vi "R45_2-RT.vi"() -> ()   [LabVIEW 2016]
uses:
  control vi/controls/Faraday cup states.ctl
  control vi/controls/Aperture states.ctl
  control vi/controls/Glassman Control.ctl
  SCA/controls/GP307 cluster.ctl
  <vilib>/FPGAPlugInAG/cRIO-9074/niLvFpga_Open_cRIO-9074.vi
  <vilib>/Utility/error.llb/Error Cluster From Error Code.vi
  <vilib>/rvi/errors/niLvFpgaAdjustHostInterfaceError.vi
  <vilib>/functionblocks/Control/PID/PID.vi
  <vilib>/rvi/interface/nirviOpenFPGA/nirviOpenFPGA.xnode
  Builds/cRIOs/R45-2-cRIO/FPGA/Controlsoftware2_FPGATarget8_R45crio2fpga_v8BgrifJ-aU.lvbitx
  R45_2-FPGA.vi
  <vilib>/rvi/interface/nirviReadWriteControl/nirviReadWriteControl.xnode
  control vi/controls/Glassman Readback.ctl
  control vi/controls/Aperture Readback.ctl
  control vi/controls/Faraday Cup Readback.ctl
  <vilib>/functionblocks/FB Core/FB Core.xnode
  <vilib>/functionblocks/NI_FunctionBlock Libraries.lvlib
  NiFpgaLv.dll
  <vilib>/NI_Real-Time Target Support.lvlib
panel:
  in  "Tab Control":T1(tab)
  out "R45 ExB 1 voltage set":dbl
  out "ExB 1- I read":dbl
  out "ExB 1- V read":dbl
  out "ExB 2+ I read":dbl
  out "ExB 2+ V read":dbl
  out "ExB 2- I read":dbl
  out "ExB 2- V read":dbl
  out "R45 ExB 2 voltage set":dbl
  out "ExB 1+ I read":dbl
  out "ExB 1+ V read":dbl
  out "GFM magnet current set":dbl
  out "GFM read string":string
  in  "output high - GFM":dbl=205.0
  in  "output low - GFM":dbl
  out "GFM field read":u8[](array[numeric])
  out "GFM field":dbl format="%#_8f"
  out "GFM command":u8[](array[numeric])
  out "R45 ExB 2 command string":string
  out "R45 ExB 2 command array":u8[](array[numeric])
  out "ExB #2 magnet current set":dbl
  out "GFM command string":string
  out "GFM field set":dbl
  out "ExB #1 magnet current set":dbl
  out "R45 ExB 1 command string":string
  out "R45 ExB 1 command array":u8[](array[numeric])
  out "proportional gain (Kc) - GFM":dbl
  out "integral time (Ti, min) - GFM":dbl
  out "derivative time (Td, min) - GFM":dbl
  out "Ion Gauge 3-2":u8[](array[numeric])
  out "Convectron gauge 3-2":u8[](array[numeric])
  out "Ion gauge 2-2":u8[](array[numeric])
  out "Ion gauge 2-1":u8[](array[numeric])
  out "Convectron 3-1":u8[](array[numeric])
  out "Ion gauge 3-1":u8[](array[numeric])
  out "Convectron 2-2":u8[](array[numeric])
  out "Convectron 2-1":u8[](array[numeric])
  out "Ion Gauge 4-1":u8[](array[numeric])
  out "Convectron Gauge 4-1":u8[](array[numeric])
  out "Ion Gauge 4-2":u8[](array[numeric])
  out "Convectron Gauge 4-2":u8[](array[numeric])
  out "R45 Quad  vac gauge cluster":T2
  out "R45 Detector vac gauge cluster":T2
  out "R45 ExB Slot vac gauge cluster":T2
  out "Detector FC status":T3
  out "Detector Aperture status":T4
  out "Detector Aperture Position":cluster{"IN sensor":bool, "OUT sensor":bool}
  out "Detector FC Position":cluster{"IN sensor":bool, "OUT sensor":bool}
  out "R45 Detector FC insert":bool
  out "R45 Detector Aperture insert":bool
  out "HV control loop error":errorcluster
  out "HV readback loop error":errorcluster
  out "Error Reporter":errorcluster
  out "ExB 1 PS loop error":errorcluster
  out "ExB 2 PS loop error":errorcluster
  out "GFM loop error":errorcluster
  out "Vacuum readback error":errorcluster
  out "Actuator loop error":errorcluster
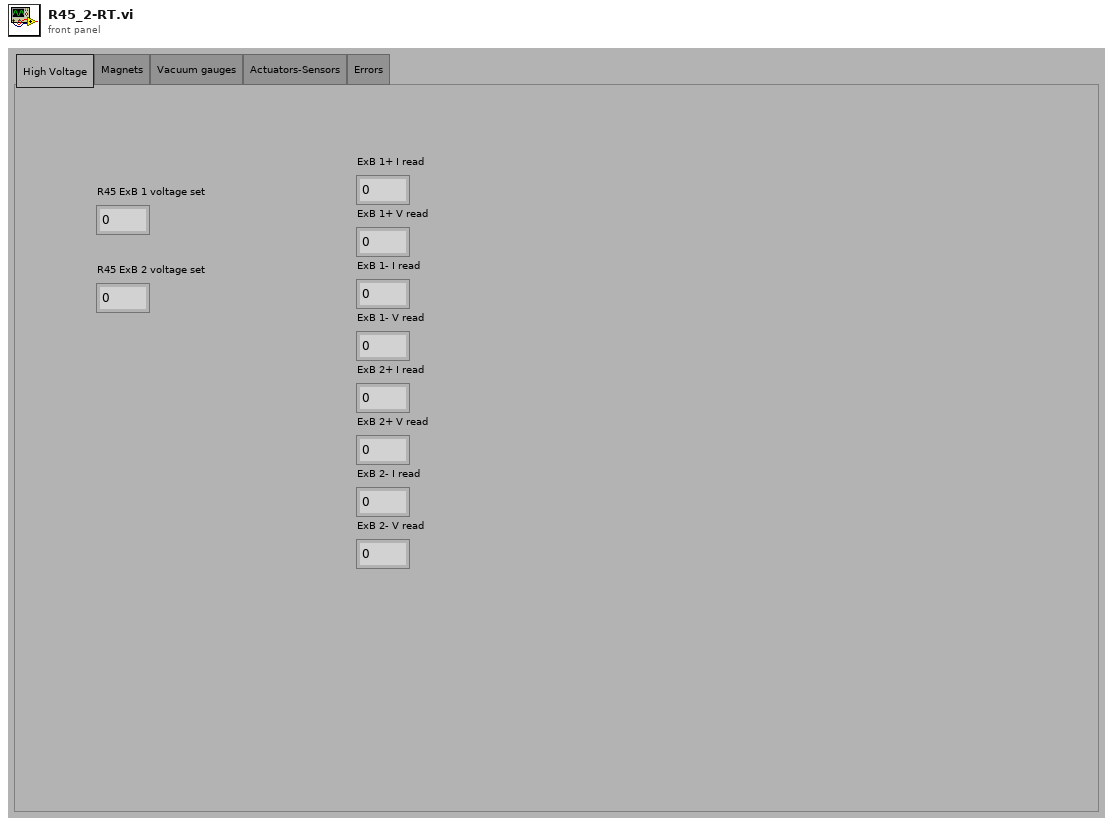
[diagram p1: front panel]
types:
  T1 = enum32{"High Voltage", "Magnets", "Vacuum gauges", "Actuators-Sensors", "Errors"}
  T2 = cluster{"Ion gauge 1":string, "Convectron  Gauge 1 ":string, "Ion Gauge 2":string, "Convectrom Gauge 2":string}
  T3 = typedef "Faraday cup states.ctl" = enum16{"FC status unclear", "FC in", "FC out"}
  T4 = typedef "Aperture states.ctl" = enum16{"Aperture status unclear", "Aperture in", "Aperture out"}
  T5 = typedef "Glassman Control.ctl" = cluster{"V-program":fxp<+/-,16,5>, "HV Enable":bool}
  T6 = typedef "Glassman Readback.ctl" = cluster{"I-monitor":fxp<+/-,16,5>, "V-monitor":fxp<+/-,16,5>}
  T7 = typedef "Aperture Readback.ctl" = cluster{"IN sensor":bool, "OUT sensor":bool}
  T8 = typedef "Faraday Cup Readback.ctl" = cluster{"IN sensor":bool, "OUT sensor":bool}
  T9 = typedef "GP307 cluster.ctl" = cluster{"Ion gauge 1":string, "Convectron  Gauge 1 ":string, "Ion Gauge 2":string, "Convectrom Gauge 2":string}
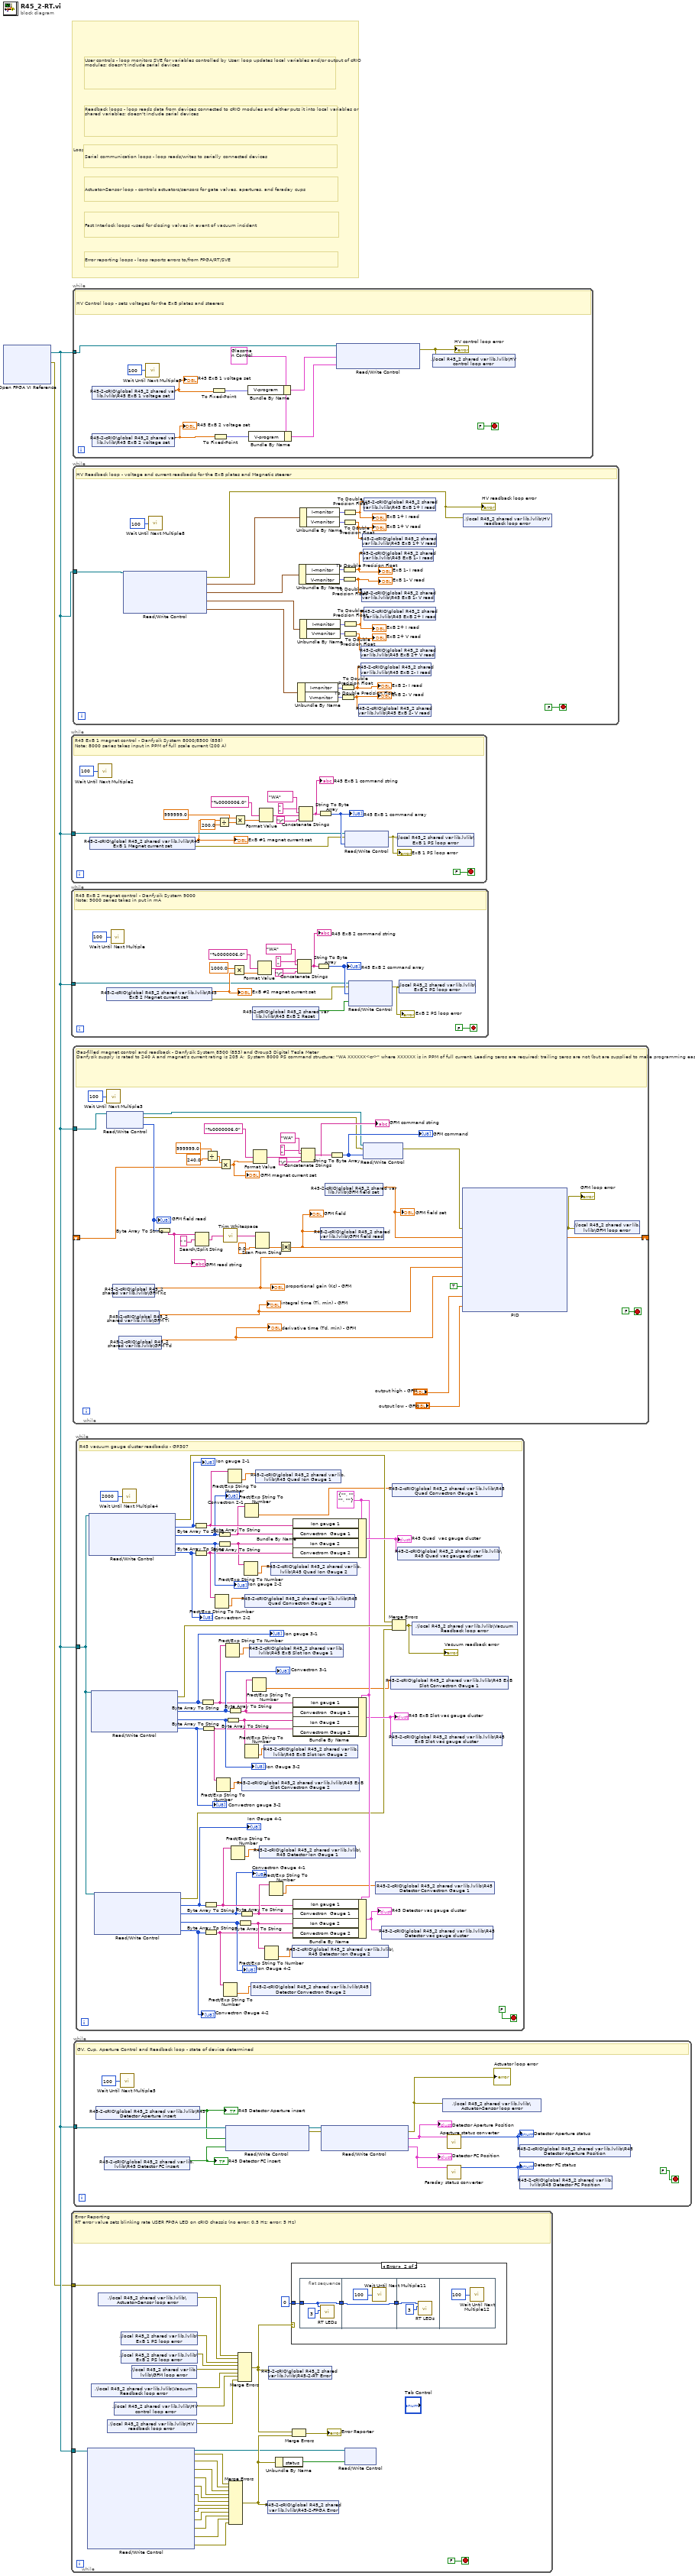
[diagram p0: block diagram]
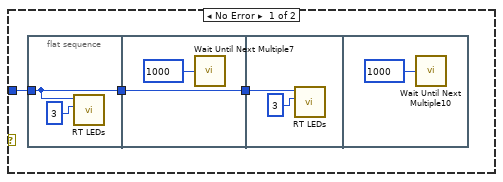
[diagram p2: hidden frame]
diagram:
  # "Serial communication loops - loop reads/writes to serially connected devices"
  # "Actuator-Sensor loop - controls actuators/sensors for gate valves, apertures, and faraday cups"
  # "Fast Interlock loops -used for closing valves in event of vacuum incident"
  # "Error reporting loops - loop reports errors to/from FPGA/RT/SVE"
  # "Readback loops - loop reads data from devices connected to cRIO modules and either puts it into local variables or shared variables; doesn't include serial devices"
  # "User controls - loop monitors SVE for variables controlled by User; loop updates local variables and/or output of cRIO modules; doesn't include serial devices"
  # "Loop legend - loops are color coded by responsibility"
  n1 = xnode "Open FPGA VI Reference"() -> ("FPGA VI Reference Out"=w2:refnum<k20>, "error out"=w1:errorcluster)  [unwired: 2 in]
  n2 = while {
    tunnel: w2 -> [w11]
    stop <- FALSE stop-if-true
    # "R45 ExB 1 magnet control - Danfysik System 8000/8500 (858)\nNote: 8000 series takes input in PPM of full scale current (200 A)"
    n3 = shared-variable "R45-2-cRIO\\global R45_2 shared var lib.lvlib\\R45 ExB 1 Magnet current set"() -> (w6:dbl, error out=w12:errorcluster)  [unwired: 1 in]
    "ExB #1 magnet current set" <- w6
    n4 = call "Wait Until Next Multiple2"("Count(mSec)"=u32 100 ("millisecond multiple")) -> ()  [unwired: 1 out]
    n5 = Divide(x=w6, y=200.0) -> (x/y=w4:dbl)
    n6 = Multiply(x=999999.0, y=w4) -> (x*y=w7:dbl)
    n7 = Format Value(format string="%0000006.0", value (0)=w7) -> (output string=w16:string)  [unwired: 1 out]
    n8 = Concatenate Strings("WA", " ", w16, "\r") -> (w18:string)
    "R45 ExB 1 command string" <- w18
    n9 = String To Byte Array(string=w18) -> (unsigned byte array=w17:u8[])
    "R45 ExB 1 command array" <- w17
    n10 = xnode "Read/Write Control"("FPGA VI Reference In"=w11, "error in"=w12, "ExB 1 PS set"=w17) -> ("error out"=w9:errorcluster)  [unwired: 1 out]
    "ExB 1 PS loop error" <- w9
    n11 = shared-variable ".\\local R45_2 shared var lib.lvlib\\ExB 1 PS loop error"(w9) -> ()  [unwired: 1 in, 1 out]
  }
  n12 = while {
    tunnel: w2 -> [w45]
    tunnel: w1 -> [w25]
    stop <- FALSE stop-if-true
    # "Error Reporting\nRT error value sets blinking rate USER FPGA LED on cRIO chassis (no error: 0.5 Hz; error: 5 Hz)"
    n13 = xnode "Read/Write Control"("FPGA VI Reference In"=w45) -> ("FPGA VI Reference Out"=w44:refnum<k20>, "error out"=w43:errorcluster, "ExB 1 PS error"=w42:errorcluster, "ExB 2 PS error"=w41:errorcluster, "GFM ps error"=w40:errorcluster, "GFM Hall Probe error"=w39:errorcluster, "HV Readback Loop"=w38:errorcluster, "HV Control Loop error"=w37:errorcluster, "Vacuum Gauge 2 error"=w24:errorcluster, "Vacuum Gauge 3 error"=w23:errorcluster, "Vacuum Gauge 4 error"=w22:errorcluster, "Position-Status Sensor error"=w34:errorcluster, "Cup-Aperture Control Loop Error"=w35:errorcluster)  [unwired: 1 in]
    n14 = shared-variable ".\\local R45_2 shared var lib.lvlib\\Vacuum Readback loop error"() -> (w30:errorcluster)  [unwired: 1 in, 1 out]
    n15 = shared-variable ".\\local R45_2 shared var lib.lvlib\\Actuator-Sensor loop error"() -> (w26:errorcluster)  [unwired: 1 in, 1 out]
    n16 = shared-variable ".\\local R45_2 shared var lib.lvlib\\HV readback loop error"() -> (w32:errorcluster)  [unwired: 1 in, 1 out]
    n17 = shared-variable ".\\local R45_2 shared var lib.lvlib\\HV control loop error"() -> (w31:errorcluster)  [unwired: 1 in, 1 out]
    n18 = shared-variable ".\\local R45_2 shared var lib.lvlib\\ExB 1 PS loop error"() -> (w27:errorcluster)  [unwired: 1 in, 1 out]
    n19 = shared-variable ".\\local R45_2 shared var lib.lvlib\\ExB 2 PS loop error"() -> (w28:errorcluster)  [unwired: 1 in, 1 out]
    n20 = shared-variable ".\\local R45_2 shared var lib.lvlib\\GFM loop error"() -> (w29:errorcluster)  [unwired: 1 in, 1 out]
    n21 = Merge Errors(w43, w42, w41, w40, w39, w38, w37, w24, w23, w22, w34, w35) -> (w47:errorcluster)
    n22 = Merge Errors(w25, w26, w27, w28, w29, w30, w31, w32) -> (w20:errorcluster)
    n23 = shared-variable "R45-2-cRIO\\global R45_2 shared var lib.lvlib\\R45-2-FPGA Error"(w47) -> ()  [unwired: 1 in, 1 out]
    n24 = shared-variable "R45-2-cRIO\\global R45_2 shared var lib.lvlib\\R45-2-RT Error"(w20) -> ()  [unwired: 1 in, 1 out]
    n25 = Unbundle By Name(w47) -> ("status"=w46:bool)
    n26 = case shown="Error" w20 {
      tunnel: 0 -> [w50 w58]
      frame No Error {
        n27 = flat-sequence {
          tunnel: w50 -> [w51]
          tunnel: [w51] -> w48
          tunnel: [w53] -> w49
          tunnel: w48 -> [w53]
          tunnel: w49 -> [w55]
          frame #0 {
            n28 = call <vilib>:"RT LEDs.vi"("State"=3, "LED Num"=w51) -> ()  [unwired: 4 in, 2 out]
          }
          frame #1 {
            n29 = call "Wait Until Next Multiple7"("Count(mSec)"=u16 1000) -> ()  [unwired: 1 out]
          }
          frame #2 {
            n30 = call <vilib>:"RT LEDs.vi"("State"=3, "LED Num"=w55) -> ()  [unwired: 4 in, 2 out]
          }
          frame #3 {
            n31 = call "Wait Until Next Multiple10"("Count(mSec)"=u16 1000) -> ()  [unwired: 1 out]
          }
        }
      }
      frame Error {
        n32 = flat-sequence {
          tunnel: [w61] -> w60
          tunnel: w58 -> [w61]
          tunnel: w60 -> [w63]
          tunnel: [w63] -> w59
          tunnel: w59 -> [w65]
          frame #0 {
            n33 = call <vilib>:"RT LEDs.vi"("State"=3, "LED Num"=w61) -> ()  [unwired: 4 in, 2 out]
          }
          frame #1 {
            n34 = call "Wait Until Next Multiple11"("Count(mSec)"=u16 100) -> ()  [unwired: 1 out]
          }
          frame #2 {
            n35 = call <vilib>:"RT LEDs.vi"("State"=3, "LED Num"=w65) -> ()  [unwired: 4 in, 2 out]
          }
          frame #3 {
            n36 = call "Wait Until Next Multiple12"("Count(mSec)"=u16 100) -> ()  [unwired: 1 out]
          }
        }
      }
    }
    n37 = Merge Errors(w20, w47) -> (→"Error Reporter":errorcluster)
    n38 = xnode "Read/Write Control"("FPGA VI Reference In"=w44, "RT error"=w46) -> ()  [unwired: 1 in, 2 out]
  }
  n39 = while {
    tunnel: w2 -> [w72]
    stop <- FALSE stop-if-true
    # "R45 ExB 2 magnet control - Danfysik System 9000\nNote: 9000 series takes in put in mA"
    n40 = shared-variable "R45-2-cRIO\\global R45_2 shared var lib.lvlib\\R45 ExB 2 Magnet current set"() -> (w80:dbl, error out=w74:errorcluster)  [unwired: 1 in]
    "ExB #2 magnet current set" <- w80
    n41 = call "Wait Until Next Multiple"("Count(mSec)"=u32 100 ("millisecond multiple")) -> ()  [unwired: 1 out]
    n42 = Multiply(x=1000.0, y=w80) -> (x*y=w69:dbl)
    n43 = shared-variable "R45-2-cRIO\\global R45_2 shared var lib.lvlib\\R45 ExB 2 Reset"() -> (w83:bool)  [unwired: 1 in, 1 out]
    n44 = Format Value(format string="%0000006.0", value (0)=w69) -> (output string=w78:string)  [unwired: 1 out]
    n45 = Concatenate Strings("WA", " ", w78, "\r") -> (w81:string)
    "R45 ExB 2 command string" <- w81
    n46 = String To Byte Array(string=w81) -> (unsigned byte array=w79:u8[])
    "R45 ExB 2 command array" <- w79
    n47 = xnode "Read/Write Control"("FPGA VI Reference In"=w72, "error in"=w74, "ExB 2 PS set"=w79, "ExB 2 Reset"=w83) -> ("error out"=w73:errorcluster)  [unwired: 1 out]
    "ExB 2 PS loop error" <- w73
    n48 = shared-variable ".\\local R45_2 shared var lib.lvlib\\ExB 2 PS loop error"(w73) -> ()  [unwired: 1 in, 1 out]
  }
  n49 = while {
    tunnel: w2 -> [w94]
    stop <- FALSE stop-if-true
    w92 = T5 {"V-program"=0.0, "HV Enable"=FALSE} ("Glassman Control")
    # "HV Control loop - sets voltages for the ExB plates and steerers"
    n50 = shared-variable "R45-2-cRIO\\global R45_2 shared var lib.lvlib\\R45 ExB 1 voltage set"() -> (w90:dbl)  [unwired: 1 in, 1 out]
    "R45 ExB 1 voltage set" <- w90
    n51 = shared-variable "R45-2-cRIO\\global R45_2 shared var lib.lvlib\\R45 ExB 2 voltage set"() -> (w88:dbl)  [unwired: 1 in, 1 out]
    "R45 ExB 2 voltage set" <- w88
    n52 = call "Wait Until Next Multiple9"("Count(mSec)"=u32 100 ("millisecond multiple")) -> ()  [unwired: 1 out]
    n53 = To Fixed-Point(number=w90) -> (fixed-point=w89:fxp<+/-,20,5>)  [unwired: 1 in]
    n54 = To Fixed-Point(number=w88) -> (fixed-point=w87:fxp<+/-,20,5>)  [unwired: 1 in]
    n55 = Bundle By Name(cluster=w92, "V-program"=w89) -> (w91:T5)
    n56 = Bundle By Name(cluster=w92, "V-program"=w87) -> (w93:T5)
    n57 = xnode "Read/Write Control"("FPGA VI Reference In"=w94, "ExB 1 - Voltage Set"=w91, "ExB 2 - Voltage Set"=w93) -> ("error out"=w86:errorcluster)  [unwired: 1 in, 1 out]
    "HV control loop error" <- w86
    n58 = shared-variable ".\\local R45_2 shared var lib.lvlib\\HV control loop error"(w86) -> ()  [unwired: 1 in, 1 out]
  }
  n59 = while {
    tunnel: w2 -> [w118]
    stop <- FALSE stop-if-true
    # "HV Readback loop - voltage and current readbacks for the ExB plates and Magnetic steerer"
    n60 = xnode "Read/Write Control"("FPGA VI Reference In"=w118) -> ("error out"=w103:errorcluster, "ExB 1+ Monitor"=w117:T6, "ExB 1- Monitor"=w116:T6, "ExB 2+ Monitor"=w115:T6, "ExB 2- Monitor"=w114:T6)  [unwired: 1 in, 1 out]
    "HV readback loop error" <- w103
    n61 = call "Wait Until Next Multiple8"("Count(mSec)"=u32 100 ("millisecond multiple")) -> ()  [unwired: 1 out]
    n62 = Unbundle By Name(w114) -> ("I-monitor"=w108:fxp<+/-,16,5>, "V-monitor"=w107:fxp<+/-,16,5>)
    n63 = Unbundle By Name(w116) -> ("I-monitor"=w112:fxp<+/-,16,5>, "V-monitor"=w111:fxp<+/-,16,5>)
    n64 = Unbundle By Name(w117) -> ("I-monitor"=w106:fxp<+/-,16,5>, "V-monitor"=w113:fxp<+/-,16,5>)
    n65 = Unbundle By Name(w115) -> ("I-monitor"=w110:fxp<+/-,16,5>, "V-monitor"=w109:fxp<+/-,16,5>)
    n66 = To Double Precision Float(number=w108) -> (double precision float=w97:dbl)
    "ExB 2- I read" <- w97
    n67 = To Double Precision Float(number=w107) -> (double precision float=w96:dbl)
    "ExB 2- V read" <- w96
    n68 = To Double Precision Float(number=w112) -> (double precision float=w101:dbl)
    "ExB 1- I read" <- w101
    n69 = To Double Precision Float(number=w111) -> (double precision float=w100:dbl)
    "ExB 1- V read" <- w100
    n70 = To Double Precision Float(number=w106) -> (double precision float=w104:dbl)
    "ExB 1+ I read" <- w104
    n71 = To Double Precision Float(number=w113) -> (double precision float=w105:dbl)
    "ExB 1+ V read" <- w105
    n72 = To Double Precision Float(number=w110) -> (double precision float=w99:dbl)
    "ExB 2+ I read" <- w99
    n73 = To Double Precision Float(number=w109) -> (double precision float=w98:dbl)
    "ExB 2+ V read" <- w98
    n74 = shared-variable "R45-2-cRIO\\global R45_2 shared var lib.lvlib\\R45 ExB 2- V read"(w96) -> ()  [unwired: 1 in, 1 out]
    n75 = shared-variable "R45-2-cRIO\\global R45_2 shared var lib.lvlib\\R45 ExB 2+ V read"(w98) -> ()  [unwired: 1 in, 1 out]
    n76 = shared-variable "R45-2-cRIO\\global R45_2 shared var lib.lvlib\\R45 ExB 2- I read"(w97) -> ()  [unwired: 1 in, 1 out]
    n77 = shared-variable "R45-2-cRIO\\global R45_2 shared var lib.lvlib\\R45 ExB 1- V read"(w100) -> ()  [unwired: 1 in, 1 out]
    n78 = shared-variable "R45-2-cRIO\\global R45_2 shared var lib.lvlib\\R45 ExB 1+ V read"(w105) -> ()  [unwired: 1 in, 1 out]
    n79 = shared-variable "R45-2-cRIO\\global R45_2 shared var lib.lvlib\\R45 ExB 1- I read"(w101) -> ()  [unwired: 1 in, 1 out]
    n80 = shared-variable "R45-2-cRIO\\global R45_2 shared var lib.lvlib\\R45 ExB 1+ I read"(w104) -> ()  [unwired: 1 in, 1 out]
    n81 = shared-variable "R45-2-cRIO\\global R45_2 shared var lib.lvlib\\R45 ExB 2+ I read"(w99) -> ()  [unwired: 1 in, 1 out]
    n82 = shared-variable ".\\local R45_2 shared var lib.lvlib\\HV readback loop error"(w103) -> ()  [unwired: 1 in, 1 out]
  }
  n83 = while {
    tunnel: w2 -> [w144]
    shift-right: [w139] -> _
    shift-left: _ -> [w134]
    stop <- FALSE stop-if-true
    # "Gas-filled magnet control and readback - Danfysik System 8500 (853) and Group3 Digital Tesla Meter\nDanfysik supply is rated to 240 A and magnet's current rating is 205 A;  System 8000 PS command structure: \"WA XXXXXX<cr>\" where XXXXXX is in PPM of full current. Leading zeros are required; trailing zeros are not (but are supplied to make programming easier)"
    n84 = call "Wait Until Next Multiple3"("Count(mSec)"=u32 100 ("millisecond multiple")) -> ()  [unwired: 1 out]
    n85 = xnode "Read/Write Control"("FPGA VI Reference In"=w144) -> ("FPGA VI Reference Out"=w143:refnum<k20>, "error out"=w142:errorcluster, "GFM read"=w145:u8[])  [unwired: 1 in]
    "GFM field read" <- w145
    n86 = shared-variable "R45-2-cRIO\\global R45_2 shared var lib.lvlib\\GFM Kc"() -> (w119:dbl)  [unwired: 1 in, 1 out]
    "proportional gain (Kc) - GFM" <- w119
    n87 = shared-variable "R45-2-cRIO\\global R45_2 shared var lib.lvlib\\GFM Ti"() -> (w137:dbl)  [unwired: 1 in, 1 out]
    "integral time (Ti, min) - GFM" <- w137
    n88 = shared-variable "R45-2-cRIO\\global R45_2 shared var lib.lvlib\\GFM Td"() -> (w136:dbl)  [unwired: 1 in, 1 out]
    "derivative time (Td, min) - GFM" <- w136
    n89 = Byte Array To String(unsigned byte array=w145) -> (string=w123:string)
    "GFM read string" <- w123
    n90 = Search/Split String(string=w123, search string/char (-)=" ") -> (match + rest of string=w121:string)  [unwired: 1 in, 2 out]
    n91 = Divide(x=999999.0, y=240.0) -> (x/y=w130:dbl)
    n92 = Multiply(x=w130, y=w134) -> (x*y=w131:dbl)
    "GFM magnet current set" <- w131
    n93 = call <vilib>:"Trim Whitespace.vi"("string"=w121) -> ("trimmed string"=w120:string)  [unwired: 1 in]
    n94 = Format Value(format string="%0000006.0", value (0)=w131) -> (output string=w151:string)  [unwired: 1 out]
    n95 = Scan From String(input string=w120, default 1=0.0) -> (output 1=w127:dbl)  [unwired: 3 in, 3 out]
    n96 = Absolute Value(x=w127) -> (abs(x)=w126:dbl)
    "GFM field" <- w126
    n97 = Concatenate Strings("WA", " ", w151, "\r") -> (w147:string)
    "GFM command string" <- w147
    n98 = shared-variable "R45-2-cRIO\\global R45_2 shared var lib.lvlib\\GFM field read"(w126) -> ()  [unwired: 1 in, 1 out]
    n99 = shared-variable "R45-2-cRIO\\global R45_2 shared var lib.lvlib\\GFM field set"() -> (w138:dbl)  [unwired: 1 in, 1 out]
    "GFM field set" <- w138
    n100 = String To Byte Array(string=w147) -> (unsigned byte array=w146:u8[])
    "GFM command" <- w146
    n101 = xnode "Read/Write Control"("FPGA VI Reference In"=w143, "error in"=w142, "GFM ps set"=w146) -> ("error out"=w141:errorcluster)  [unwired: 1 out]
    n102 = xnode "PID"("error in"=w141, "setpoint"=w138, "process variable"=w126, "proportional gain (Kc)"=w119, "integral time (Ti, min)"=w137, "derivative time (Td, min)"=w136, "auto? (T)"=TRUE, "output high"="output high - GFM", "output low"="output low - GFM") -> ("error out"=w140:errorcluster, "output"=w139:dbl)
    "GFM loop error" <- w140
    n103 = shared-variable ".\\local R45_2 shared var lib.lvlib\\GFM loop error"(w140) -> ()  [unwired: 1 in, 1 out]
  }
  n104 = while {
    tunnel: w2 -> [w230]
    stop <- FALSE stop-if-true
    # "GV, Cup, Aperture Control and Readback loop - state of device determined"
    n105 = shared-variable "R45-2-cRIO\\global R45_2 shared var lib.lvlib\\R45 Detector Aperture insert"() -> (w227:bool)  [unwired: 1 in, 1 out]
    "R45 Detector Aperture insert" <- w227
    n106 = shared-variable "R45-2-cRIO\\global R45_2 shared var lib.lvlib\\R45 Detector FC insert"() -> (w226:bool)  [unwired: 1 in, 1 out]
    "R45 Detector FC insert" <- w226
    n107 = call "Wait Until Next Multiple5"("Count(mSec)"=u32 100 ("millisecond multiple")) -> ()  [unwired: 1 out]
    n108 = xnode "Read/Write Control"("FPGA VI Reference In"=w230, "Detector Aperture insert"=w227, "Detector FC insert"=w226) -> ("FPGA VI Reference Out"=w229:refnum<k20>, "error out"=w228:errorcluster)  [unwired: 1 in]
    n109 = xnode "Read/Write Control"("FPGA VI Reference In"=w229, "error in"=w228) -> ("error out"=w225:errorcluster, "Detector Aperture Position"=w222:T7, "Detector FC Position"=w224:T8)  [unwired: 1 out]
    "Detector Aperture Position" <- w222
    "Detector FC Position" <- w224
    "Actuator loop error" <- w225
    n110 = shared-variable ".\\local R45_2 shared var lib.lvlib\\Actuator-Sensor loop error"(w225) -> ()  [unwired: 1 in, 1 out]
    n111 = call "Aperture status converter.vi"("Aperture Position"=w222) -> ("Aperture Status"=w221:T4)  [unwired: 10 in]
    "Detector Aperture status" <- w221
    n112 = call "Faraday status converter.vi"("FC Position"=w224) -> ("FC Status"=w223:T3)  [unwired: 10 in]
    "Detector FC status" <- w223
    n113 = shared-variable "R45-2-cRIO\\global R45_2 shared var lib.lvlib\\R45 Detector Aperture Position"(w221) -> ()  [unwired: 1 in, 1 out]
    n114 = shared-variable "R45-2-cRIO\\global R45_2 shared var lib.lvlib\\R45 Detector FC Position"(w223) -> ()  [unwired: 1 in, 1 out]
  }
  n115 = while {
    tunnel: w2 -> [w256]
    stop <- FALSE stop-if-true
    w267 = T9 {"Ion gauge 1"="", "Convectron  Gauge 1 "="", "Ion Gauge 2"="", "Convectrom Gauge 2"=""} ("Ion gauge cluster control")
    # "R45 vacuum gauge cluster readbacks - GP307"
    n116 = xnode "Read/Write Control"("FPGA VI Reference In"=w256) -> ("error out"=w246:errorcluster, "Vac Cluster 2 Ion Gauge 1"=w255:u8[], "Vac Cluster 2 Convectron 1"=w254:u8[], "Vac Cluster 2 Ion Gauge 2"=w253:u8[], "Vac Cluster 2 Convectron 2"=w252:u8[])  [unwired: 1 in, 1 out]
    "Ion gauge 2-1" <- w255
    "Convectron 2-1" <- w254
    "Ion gauge 2-2" <- w253
    "Convectron 2-2" <- w252
    n117 = xnode "Read/Write Control"("FPGA VI Reference In"=w256) -> ("error out"=w278:errorcluster, "Vac Cluster 3 Ion Gauge 1"=w276:u8[], "Vac Cluster 3 Convectron 1"=w275:u8[], "Vac Cluster 3 Ion Gauge 2"=w273:u8[], "Vac Cluster 3 Convectron 2"=w274:u8[])  [unwired: 1 in, 1 out]
    "Ion gauge 3-1" <- w276
    "Convectron 3-1" <- w275
    "Convectron gauge 3-2" <- w274
    "Ion Gauge 3-2" <- w273
    n118 = xnode "Read/Write Control"("FPGA VI Reference In"=w256) -> ("error out"=w245:errorcluster, "Vac Cluster 4 Ion Gauge 1"=w259:u8[], "Vac Cluster 4 Convectron 1"=w261:u8[], "Vac Cluster 4 Ion Gauge 2"=w262:u8[], "Vac Cluster 4 Convectron 2"=w260:u8[])  [unwired: 1 in, 1 out]
    "Ion Gauge 4-1" <- w259
    "Convectron Gauge 4-1" <- w261
    "Ion Gauge 4-2" <- w262
    "Convectron Gauge 4-2" <- w260
    n119 = call "Wait Until Next Multiple4"("Count(mSec)"=u32 2000 ("millisecond multiple")) -> ()  [unwired: 1 out]
    n120 = Byte Array To String(unsigned byte array=w255) -> (string=w271:string)
    n121 = Byte Array To String(unsigned byte array=w252) -> (string=w249:string)
    n122 = Byte Array To String(unsigned byte array=w276) -> (string=w270:string)
    n123 = Byte Array To String(unsigned byte array=w274) -> (string=w251:string)
    n124 = Byte Array To String(unsigned byte array=w259) -> (string=w263:string)
    n125 = Byte Array To String(unsigned byte array=w260) -> (string=w257:string)
    n126 = Fract/Exp String To Number(string=w249) -> (number=w234:dbl)  [unwired: 3 in, 1 out]
    n127 = Fract/Exp String To Number(string=w251) -> (number=w238:dbl)  [unwired: 3 in, 1 out]
    n128 = Byte Array To String(unsigned byte array=w254) -> (string=w268:string)
    n129 = Byte Array To String(unsigned byte array=w253) -> (string=w248:string)
    n130 = Fract/Exp String To Number(string=w257) -> (number=w241:dbl)  [unwired: 3 in, 1 out]
    n131 = Fract/Exp String To Number(string=w270) -> (number=w240:dbl)  [unwired: 3 in, 1 out]
    n132 = Byte Array To String(unsigned byte array=w273) -> (string=w250:string)
    n133 = Fract/Exp String To Number(string=w271) -> (number=w236:dbl)  [unwired: 3 in, 1 out]
    n134 = Byte Array To String(unsigned byte array=w275) -> (string=w269:string)
    n135 = Fract/Exp String To Number(string=w263) -> (number=w244:dbl)  [unwired: 3 in, 1 out]
    n136 = Byte Array To String(unsigned byte array=w262) -> (string=w258:string)
    n137 = Byte Array To String(unsigned byte array=w261) -> (string=w264:string)
    n138 = shared-variable "R45-2-cRIO\\global R45_2 shared var lib.lvlib\\R45 ExB Slot Convectron Gauge 2"(w238) -> ()  [unwired: 1 in, 1 out]
    n139 = Fract/Exp String To Number(string=w248) -> (number=w235:dbl)  [unwired: 3 in, 1 out]
    n140 = Fract/Exp String To Number(string=w268) -> (number=w233:dbl)  [unwired: 3 in, 1 out]
    n141 = shared-variable "R45-2-cRIO\\global R45_2 shared var lib.lvlib\\R45 Quad Convectron Gauge 2"(w234) -> ()  [unwired: 1 in, 1 out]
    n142 = Fract/Exp String To Number(string=w250) -> (number=w239:dbl)  [unwired: 3 in, 1 out]
    n143 = shared-variable "R45-2-cRIO\\global R45_2 shared var lib.lvlib\\R45 ExB Slot Ion Gauge 1"(w240) -> ()  [unwired: 1 in, 1 out]
    n144 = shared-variable "R45-2-cRIO\\global R45_2 shared var lib.lvlib\\R45 Detector Convectron Gauge 2"(w241) -> ()  [unwired: 1 in, 1 out]
    n145 = Fract/Exp String To Number(string=w269) -> (number=w237:dbl)  [unwired: 3 in, 1 out]
    n146 = shared-variable "R45-2-cRIO\\global R45_2 shared var lib.lvlib\\R45 Quad Ion Gauge 1"(w236) -> ()  [unwired: 1 in, 1 out]
    n147 = shared-variable "R45-2-cRIO\\global R45_2 shared var lib.lvlib\\R45 Detector Ion Gauge 1"(w244) -> ()  [unwired: 1 in, 1 out]
    n148 = shared-variable "R45-2-cRIO\\global R45_2 shared var lib.lvlib\\R45 ExB Slot Ion Gauge 2"(w239) -> ()  [unwired: 1 in, 1 out]
    n149 = Fract/Exp String To Number(string=w258) -> (number=w243:dbl)  [unwired: 3 in, 1 out]
    n150 = Fract/Exp String To Number(string=w264) -> (number=w242:dbl)  [unwired: 3 in, 1 out]
    n151 = shared-variable "R45-2-cRIO\\global R45_2 shared var lib.lvlib\\R45 Quad Ion Gauge 2"(w235) -> ()  [unwired: 1 in, 1 out]
    n152 = shared-variable "R45-2-cRIO\\global R45_2 shared var lib.lvlib\\R45 Detector Ion Gauge 2"(w243) -> ()  [unwired: 1 in, 1 out]
    n153 = Bundle By Name(cluster=w267, "Ion gauge 1"=w271, "Convectron  Gauge 1"=w268, "Ion Gauge 2"=w248, "Convectrom Gauge 2"=w249) -> (w272:T9)
    "R45 Quad  vac gauge cluster" <- w272
    n154 = Bundle By Name(cluster=w267, "Ion gauge 1"=w270, "Convectron  Gauge 1"=w269, "Ion Gauge 2"=w251, "Convectrom Gauge 2"=w250) -> (w265:T9)
    "R45 ExB Slot vac gauge cluster" <- w265
    n155 = Bundle By Name(cluster=w267, "Ion gauge 1"=w263, "Convectron  Gauge 1"=w264, "Ion Gauge 2"=w258, "Convectrom Gauge 2"=w257) -> (w266:T9)
    "R45 Detector vac gauge cluster" <- w266
    n156 = shared-variable "R45-2-cRIO\\global R45_2 shared var lib.lvlib\\R45 Detector Convectron Gauge 1"(w242) -> ()  [unwired: 1 in, 1 out]
    n157 = shared-variable "R45-2-cRIO\\global R45_2 shared var lib.lvlib\\R45 Detector vac gauge cluster"(w266) -> ()  [unwired: 1 in, 1 out]
    n158 = shared-variable "R45-2-cRIO\\global R45_2 shared var lib.lvlib\\R45 ExB Slot Convectron Gauge 1"(w237) -> ()  [unwired: 1 in, 1 out]
    n159 = shared-variable "R45-2-cRIO\\global R45_2 shared var lib.lvlib\\R45 Quad Convectron Gauge 1"(w233) -> ()  [unwired: 1 in, 1 out]
    n160 = Merge Errors(w246, w278, w245) -> (w247:errorcluster)
    "Vacuum readback error" <- w247
    n161 = shared-variable "R45-2-cRIO\\global R45_2 shared var lib.lvlib\\R45 ExB Slot vac gauge cluster"(w265) -> ()  [unwired: 1 in, 1 out]
    n162 = shared-variable "R45-2-cRIO\\global R45_2 shared var lib.lvlib\\R45 Quad vac gauge cluster"(w272) -> ()  [unwired: 1 in, 1 out]
    n163 = shared-variable ".\\local R45_2 shared var lib.lvlib\\Vacuum Readback loop error"(w247) -> ()  [unwired: 1 in, 1 out]
  }
